vi "GUI_HTT_MultiCamDriveExperiment2.vi"() -> ()   [LabVIEW 2020]
uses:
  Shared/GUI_Template/GUI_master/tcp_new_data_event.ctl
  Shared/GUI_Template/GUI_master/tcp new data cluster.ctl
  General GUIs/Device GUIs/GUI_Cameras/Controls/Crosshair type def.ctl
  <userlib>/_OpenG.lib/array/array.llb/Filter 1D Array with Scalar (String)__ogtk.vi
panel:
  out "String 3":string="x1\ny1\nx2\ny2"
  out "String 2":string="x1\ny1\nx2\ny2"
  out "String":string="x1\ny1\nx2\ny2"
  in  "visibility":bool=TRUE
  out "appended array":string[](array[string]) caption="XH"
  out "appended array 6":string[](array[string]) caption="XH"
  out "appended array 4":string[](array[string]) caption="XH"
  in  "UDP error message":string
  out "tcp data event 2":T1
  out "error IO 2":errorcluster
  in  "Color Box":u32(colorbox)
  in  "TargetSize.Y::4":dbl=45.0 caption="y" min=2.0 max=3000.0 format="%#_6f"
  in  "TargetSize.X::4":dbl=47.0 caption="x" min=2.0 max=3000.0 format="%#_6f"
  in  "TargetSize.Y::3":dbl=163.0 caption="y" min=2.0 max=3000.0 format="%#_6f"
  in  "TargetSize.X::3":dbl=152.0 caption="x" min=2.0 max=3000.0 format="%#_6f"
  in  "TargetSize.Y::2":dbl=74.0 caption="y" min=2.0 max=3000.0 format="%#_6f"
  in  "TargetSize.X::2":dbl=75.0 caption="x" min=2.0 max=3000.0 format="%#_6f"
  in  "active cams":string
  out "CCDs":string[](array[string])
  out "Cameras":T2
  in  "Target.Y::4":dbl=45.0 caption="y" min=0.0 max=2000.0 format="%#_6f"
  in  "Target.X::4":dbl=47.0 caption="x" min=0.0 max=2000.0 format="%#_6f"
  in  "Target.Y::3":dbl=163.0 caption="y" min=0.0 max=2000.0 format="%#_6f"
  in  "Target.X::3":dbl=152.0 caption="x" min=0.0 max=2000.0 format="%#_6f"
  in  "Target.Y::2":dbl=74.0 caption="y" min=0.0 max=2000.0 format="%#_6f"
  in  "Target.X::2":dbl=75.0 caption="x" min=0.0 max=2000.0 format="%#_6f"
  out "error out":errorcluster
  in  "triggerdelay::4":dbl=0.001 caption="triggerdelay" min=0.0 max=10000000.0 format="%_4p"
  in  "triggerdelay::3":dbl=0.001 caption="triggerdelay" min=0.0 max=10000000.0 format="%_4p"
  in  "triggerdelay::2":dbl=0.001 caption="triggerdelay" min=0.0 max=1000000.0 format="%_4p"
  in  "centroidy::5":dbl=0.001 caption="centroid y" min=0.0 max=0.0 format="%_4f"
  in  "centroidx::5":dbl=0.001 caption="centroid x" min=0.0 max=0.0 format="%_4f"
  in  "trigger::4":bool caption="Trigger"
  in  "centroidy::4":dbl=0.001 caption="centroid y" min=0.0 max=0.0 format="%_4f"
  in  "centroidx::4":dbl=0.001 caption="centroid x" min=0.0 max=0.0 format="%_4f"
  in  "exposure::4":dbl=0.001 caption="exposure" min=0.0001 max=100000.0 format="%_4p"
  out "image::4":T3(plugin-control) caption="HTT-MagCam-02"
  in  "GUIdevice 4":string="HTT-C14_3_topjet"
  in  "trigger::3":bool caption="Trigger"
  in  "centroidy::3":dbl=0.001 caption="centroid y" min=0.0 max=0.0 format="%_4f"
  in  "centroidx::3":dbl=0.001 caption="centroid x" min=0.0 max=0.0 format="%_4f"
  in  "exposure::3":dbl=0.001 caption="exposure" min=1.0 max=10000000.0 format="%_4p"
  out "image::3":T3(plugin-control) caption="HTT-MagCam-03"
  in  "GUIdevice 3":string="HTT-C26_1_ppoint2"
  in  "trigger::2":bool caption="Trigger"
  in  "centroidy::2":dbl=0.001 caption="centroid y" min=0.0 max=0.0 format="%_4f"
  in  "centroidx::2":dbl=0.001 caption="centroid x" min=0.0 max=0.0 format="%_4f"
  in  "exposure::2":dbl=0.001 caption="exposure" min=0.0001 max=1.0 format="%_4p"
  out "image::2":T3(plugin-control) caption="HTT-MagCam-04"
  in  "GUIdevice 2":string="HTT-C14_2_if"
  out "tcp data event":T1
  in  "Refresh Button":bool caption="Update Crosshairs"
  in  "Select device":string(combo)="FrogHPD"
  in  "stop":bool
  in  "GUIdevice 1":string="HPD_CCD"
  # "XHair location"
  # "XHair location"
  # "XHair size"
  # "XHair size"
  # "XHair location"
  # "XHair size"
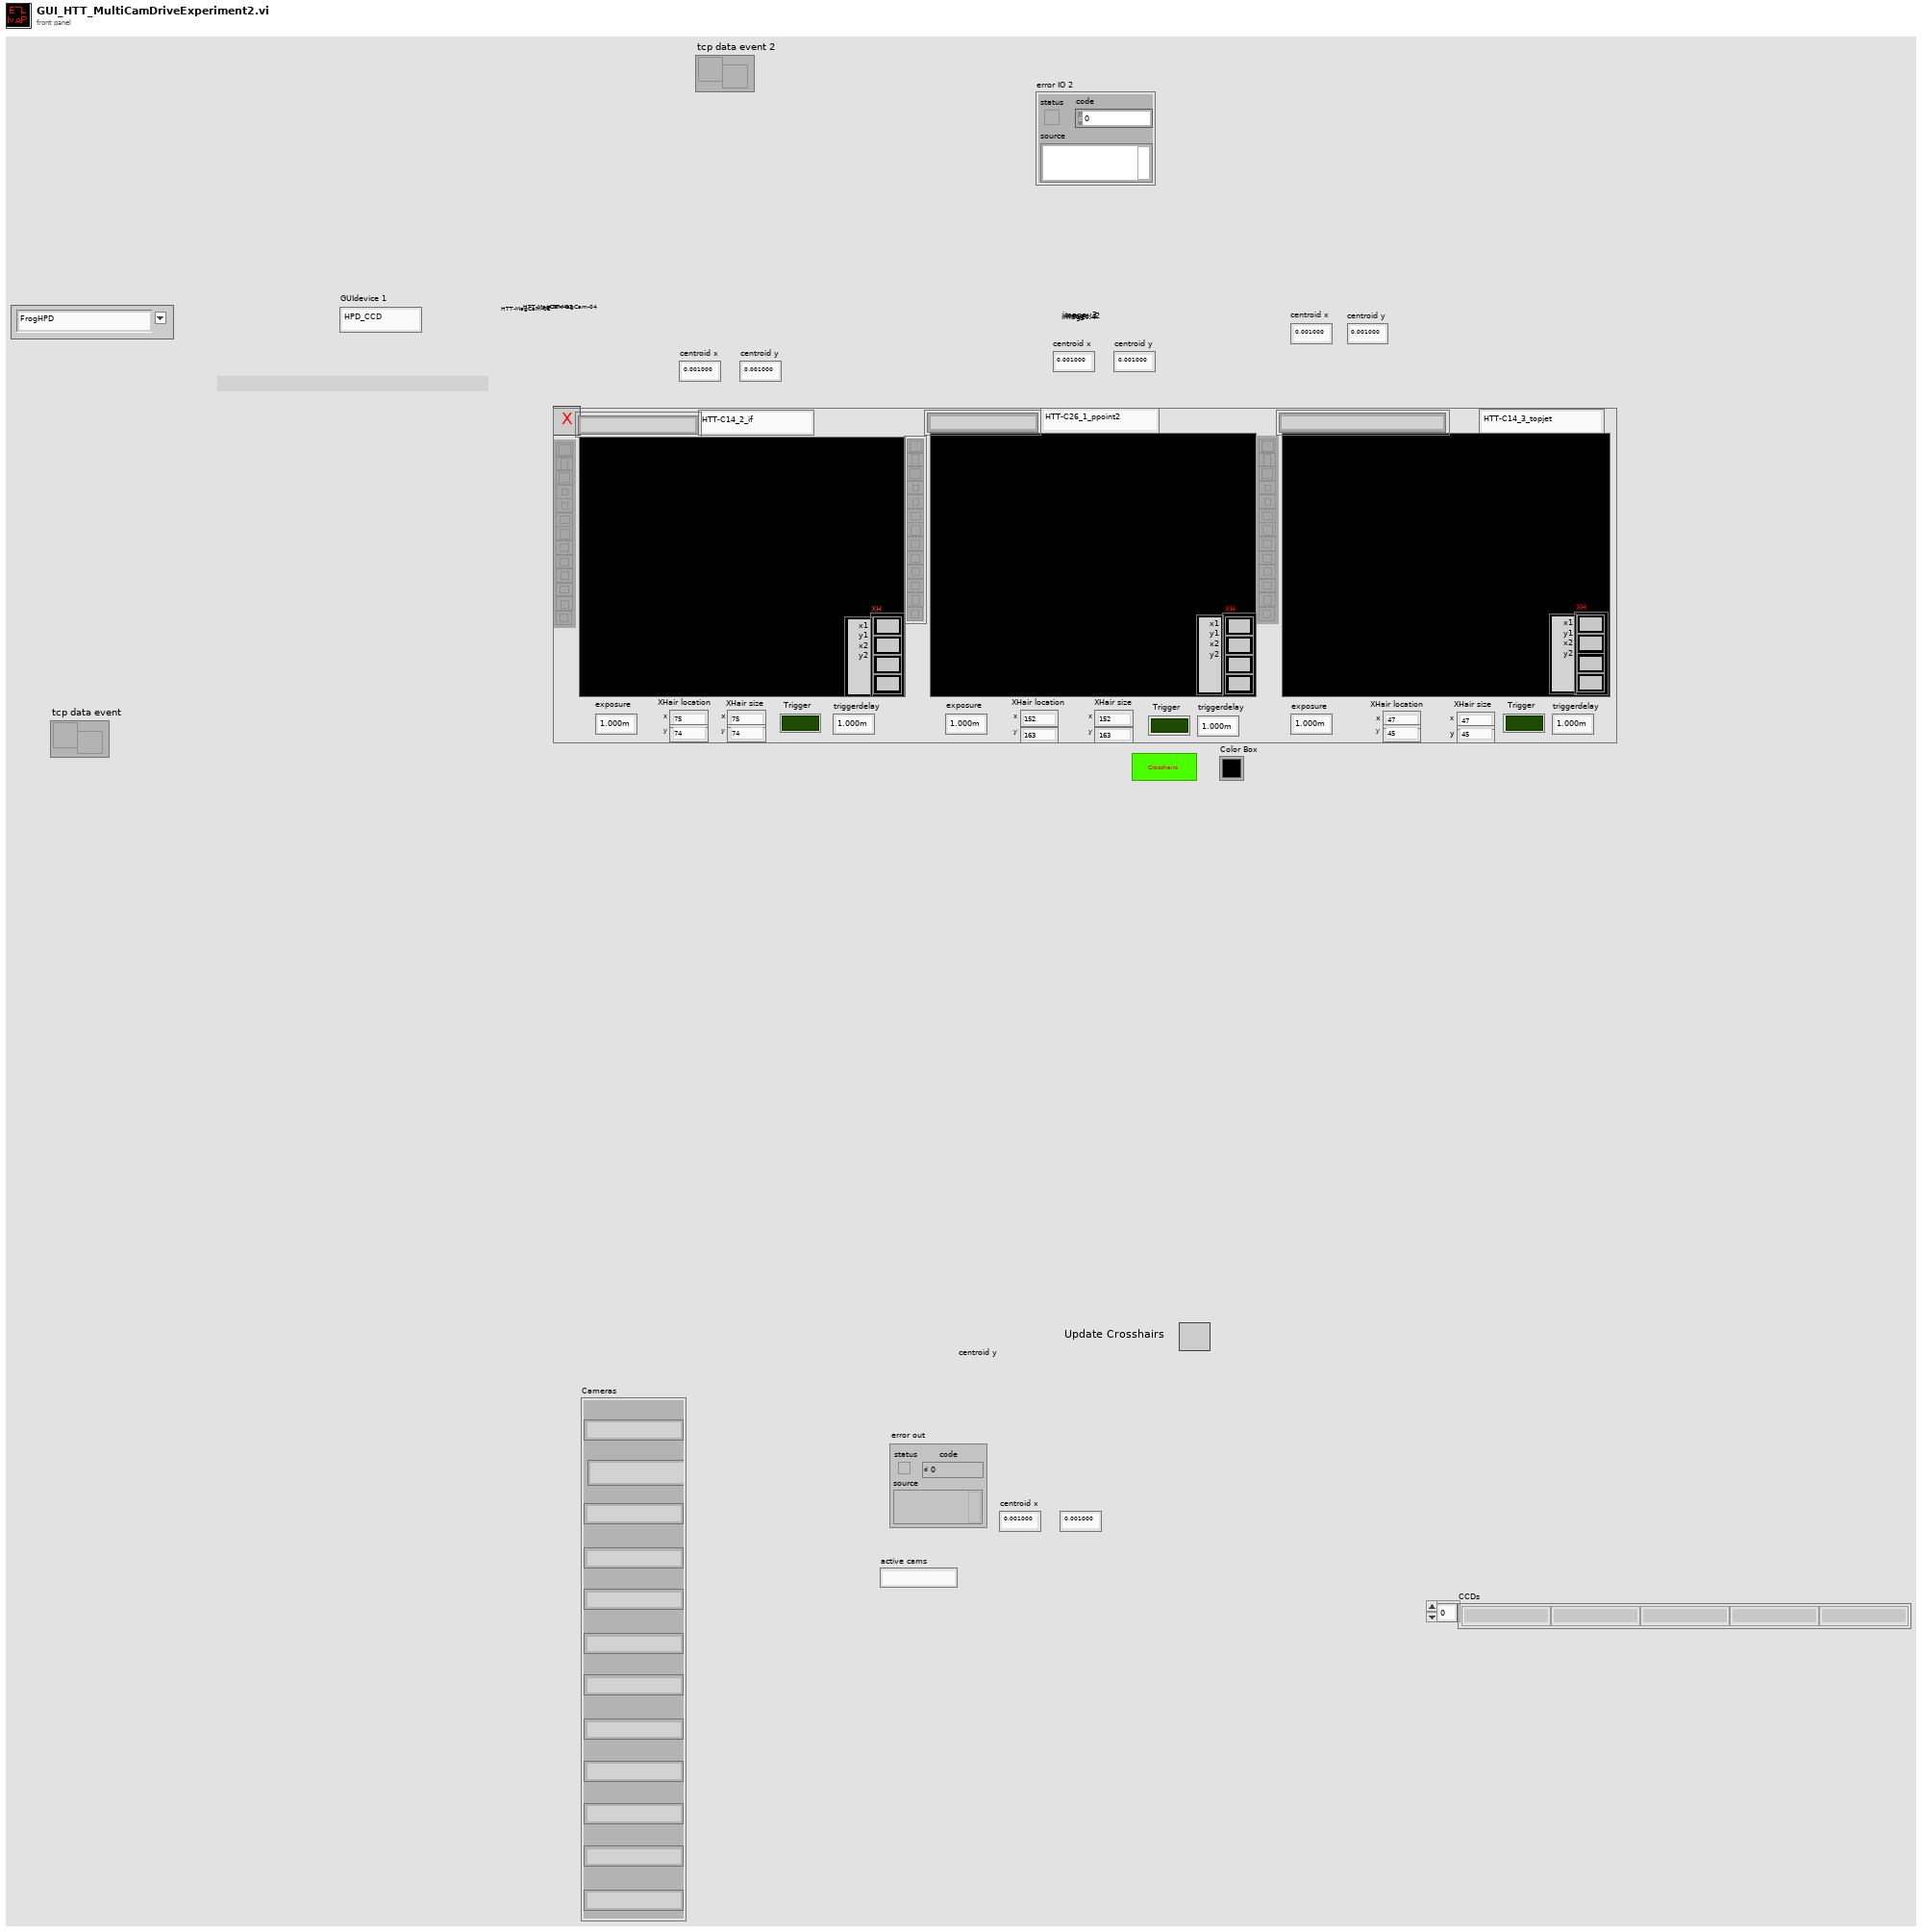
[diagram p1: front panel]
types:
  T1 = typedef "tcp_new_data_event.ctl" = refnum<user-event>
  T2 = cluster{"[0]":string, "[1]":string, "[2]":string, "[3]":string, "[4]":string, "[5]":string, "[6]":string, "[7]":string, "[8]":string, "[8] 2":string, "[8] 3":string, "[8] 4":string}
  T3 = typedef "IMAQ Image.ctl" = refnum<image>
  T4 = typedef "Image Type" = u32
  T5 = cluster{"Target.X::2":refnum<vi>, "Target.Y::2":refnum<vi>}
  T6 = cluster{"Target.X::3":refnum<vi>, "Target.Y::3":refnum<vi>}
  T7 = cluster{"Target.X::4":refnum<vi>, "Target.Y::4":refnum<vi>}
  T8 = cluster{"TargetSize.X::2":refnum<vi>, "TargetSize.Y::2":refnum<vi>}
  T9 = cluster{"TargetSize.X::3":refnum<vi>, "TargetSize.Y::3":refnum<vi>}
  T10 = cluster{"TargetSize.X::4":refnum<vi>, "TargetSize.Y::4":refnum<vi>}
  T11 = cluster{"Target.X::4":refnum<vi>, "Target.Y::4":refnum<vi>}[]
  T12 = cluster{"TargetSize.X::4":refnum<vi>, "TargetSize.Y::4":refnum<vi>}[]
  T13 = cluster{"[0]":string, "[1]":string, "[2]":string, "[3]":string, "[4]":string, "[5]":string, "[6]":string, "[7]":string, "[8]":string, "[9]":string, "[10]":string, "[11]":string}
  T14 = typedef "Crosshair type def.ctl" = cluster{"Draw":bool, "Target":cluster{"x":dbl, "y":dbl}, "Size":cluster{"x":dbl, "y":dbl}, "Angle":dbl, "Color":u32, "Thickness":u8, "CrosshairLabel":string}
  T15 = cluster{"Left":i32, "Top":i32, "Right":i32, "Bottom":i32}
  T16 = enum32{"invalid app kind", "Development System", "Run Time System", "Student Edition", "Embedded LabVIEW", "Evaluation", "Custom"}
  T17 = typedef "tcp new data cluster.ctl" = cluster{"EventEnum":enum16{"new data", "connection status update"}, "Device name":string}
  T18 = enum32{"Invalid", "Standard", "Closed", "Hidden", "Minimized", "Maximized"}
  T19 = cluster{"Core":cluster{"Current VI Reference":refnum<vi>, "Close Panel on Exit?":bool}, "Your Boolean data":bool, "active cams":string, "SuperGUI":cluster{"STOP queue":refnum<queue>, "SuperGUI ref":refnum<vi>}}
  T20 = cluster{"STOP queue":refnum<queue>, "SuperGUI ref":refnum<vi>}
  T21 = cluster{"Current VI Reference":refnum<vi>, "Close Panel on Exit?":bool}
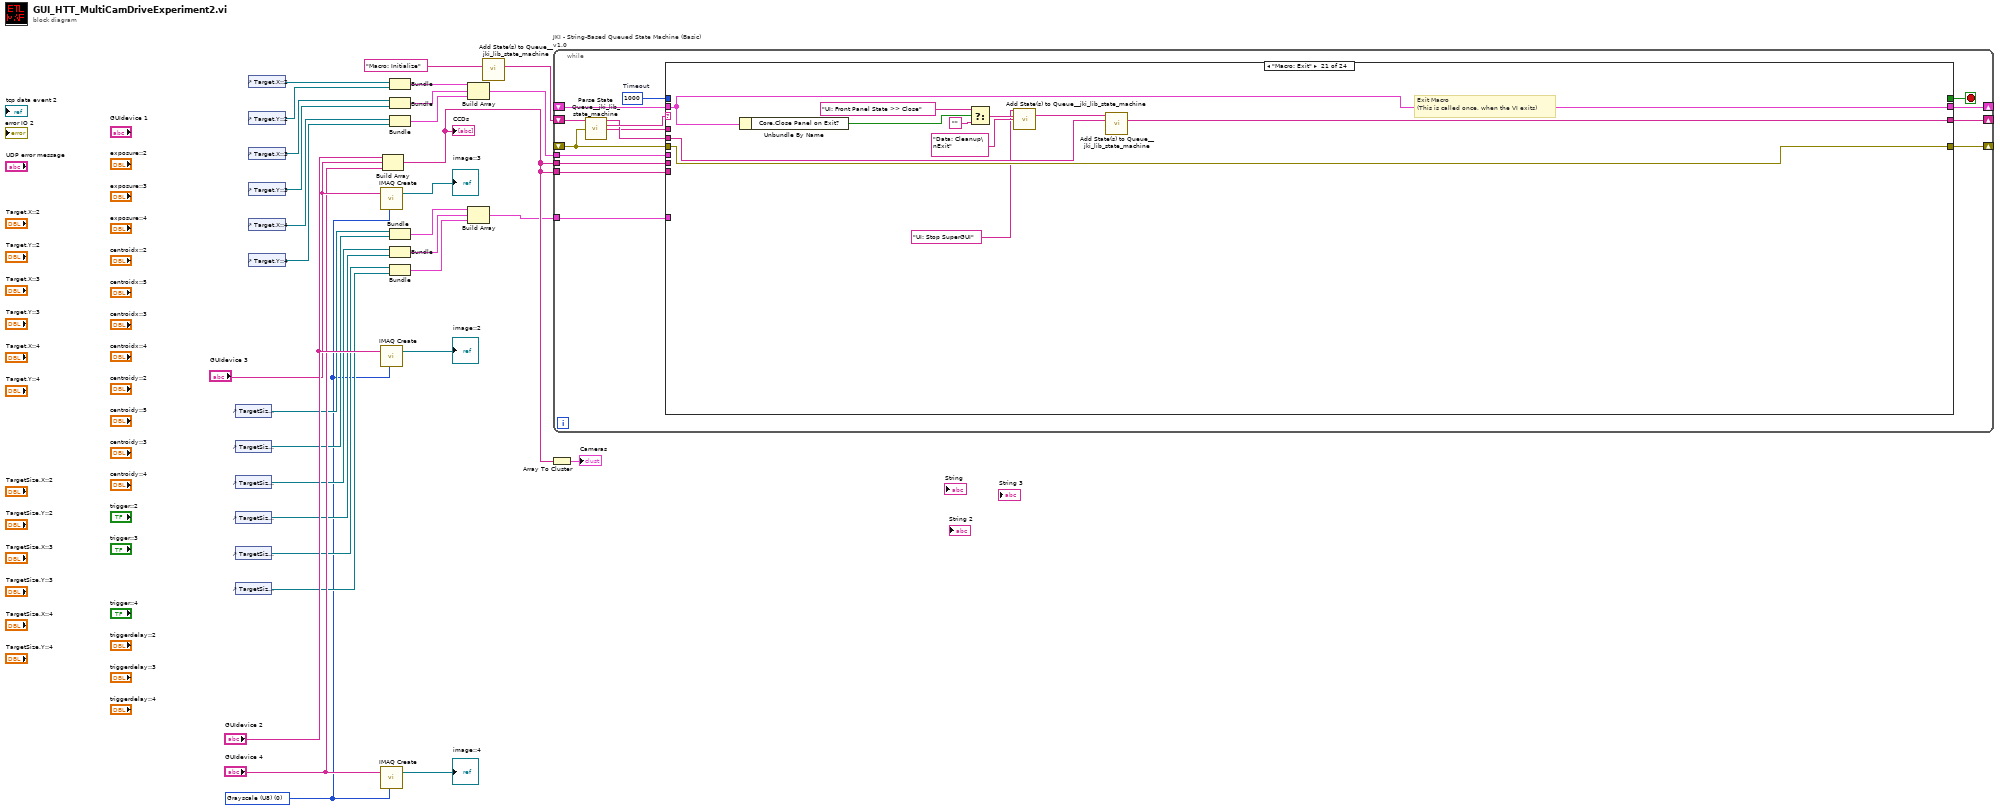
[diagram p0: block diagram]
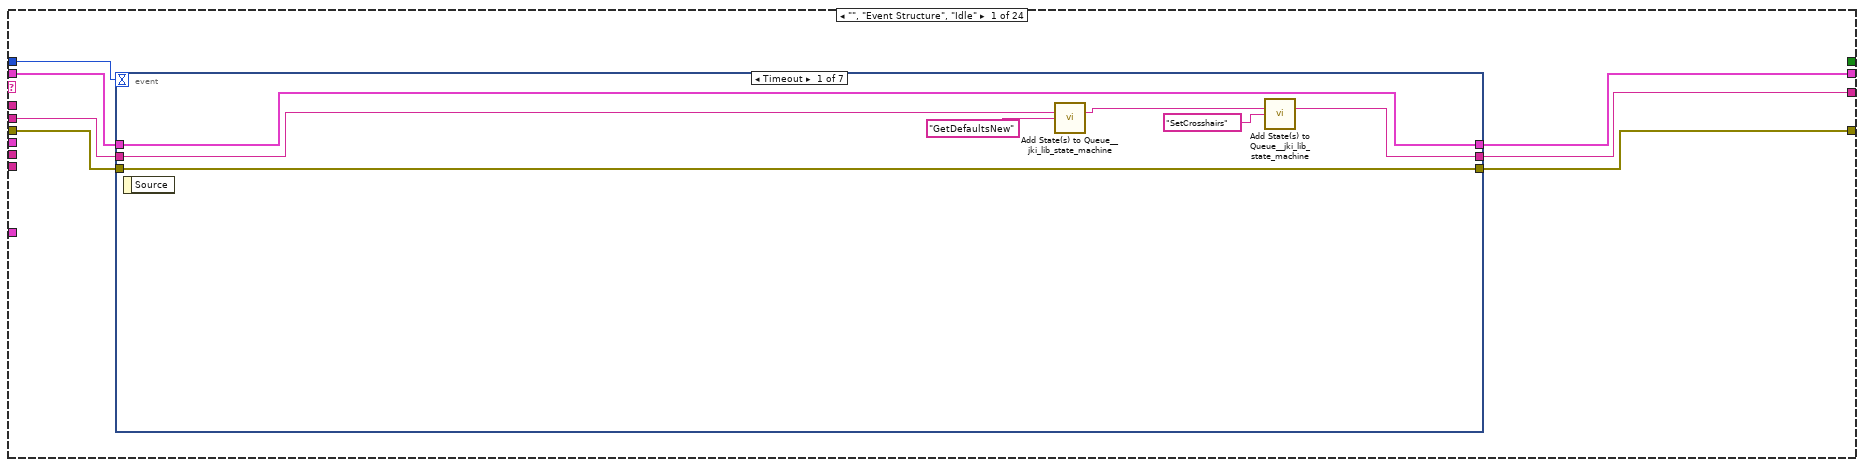
[diagram p2: hidden frame]
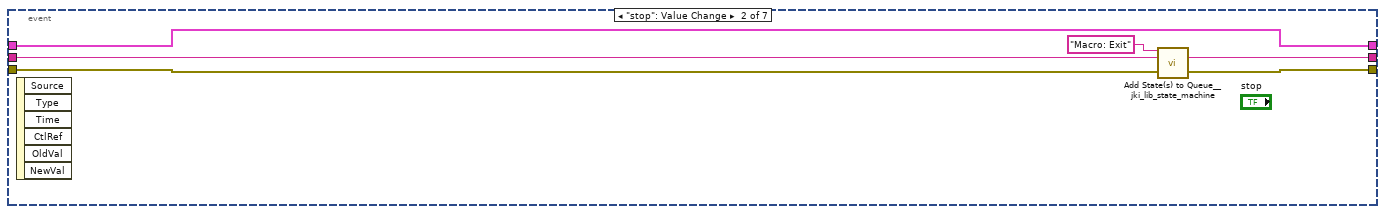
[diagram p3: hidden frame]
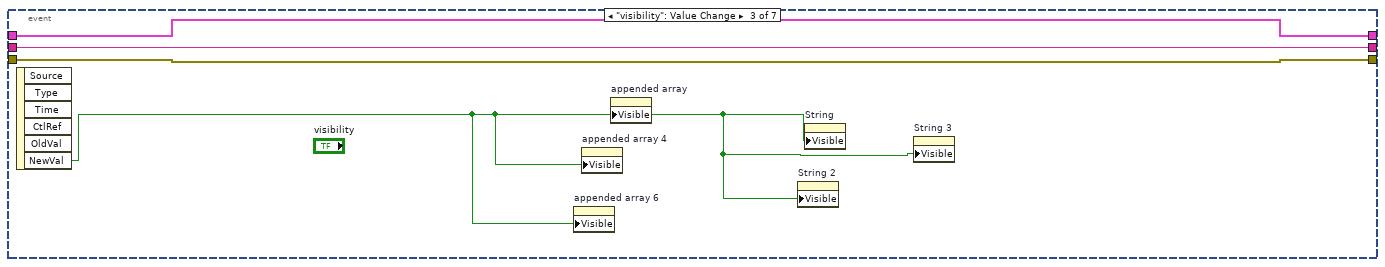
[diagram p4: hidden frame]
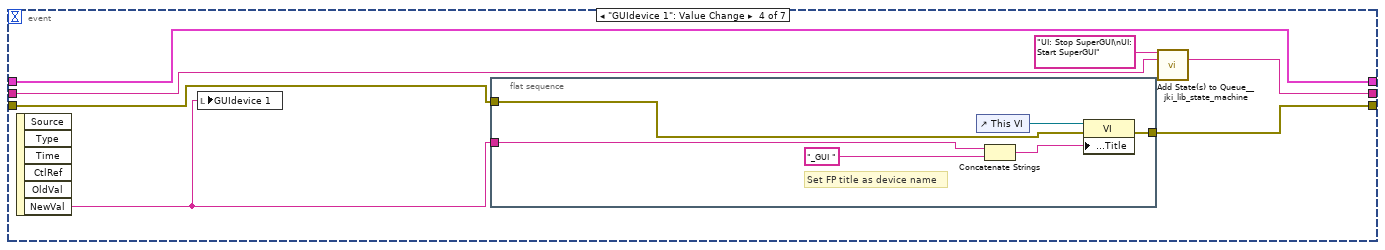
[diagram p5: hidden frame]
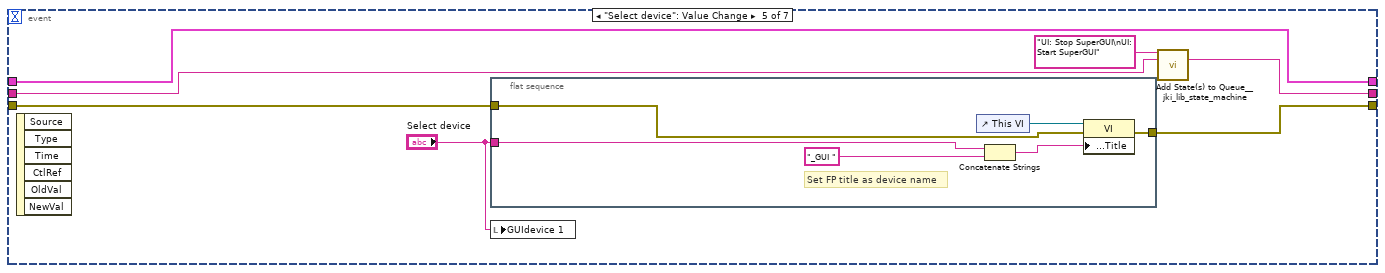
[diagram p6: hidden frame]
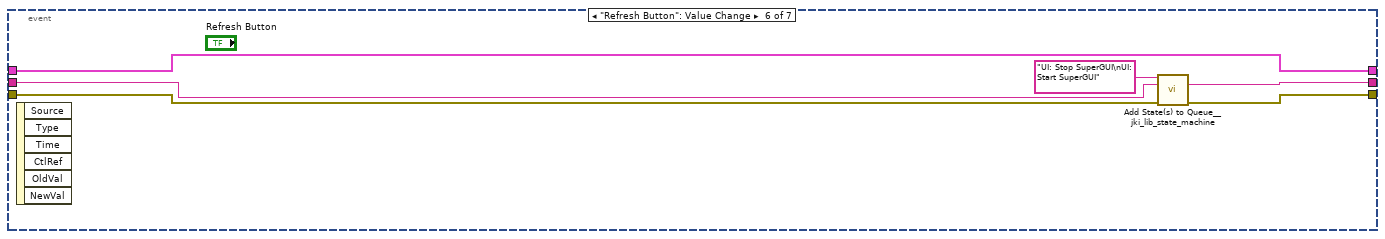
[diagram p7: hidden frame]
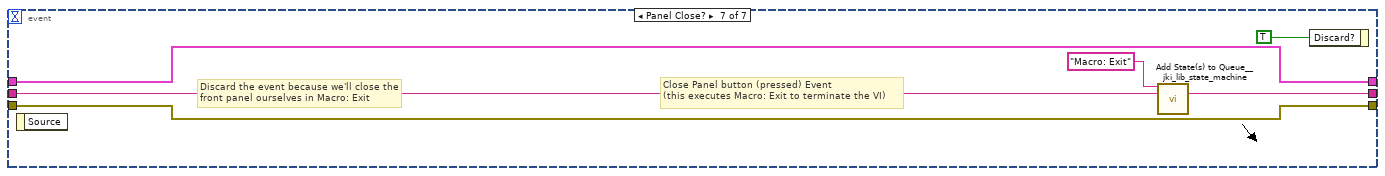
[diagram p8: hidden frame]
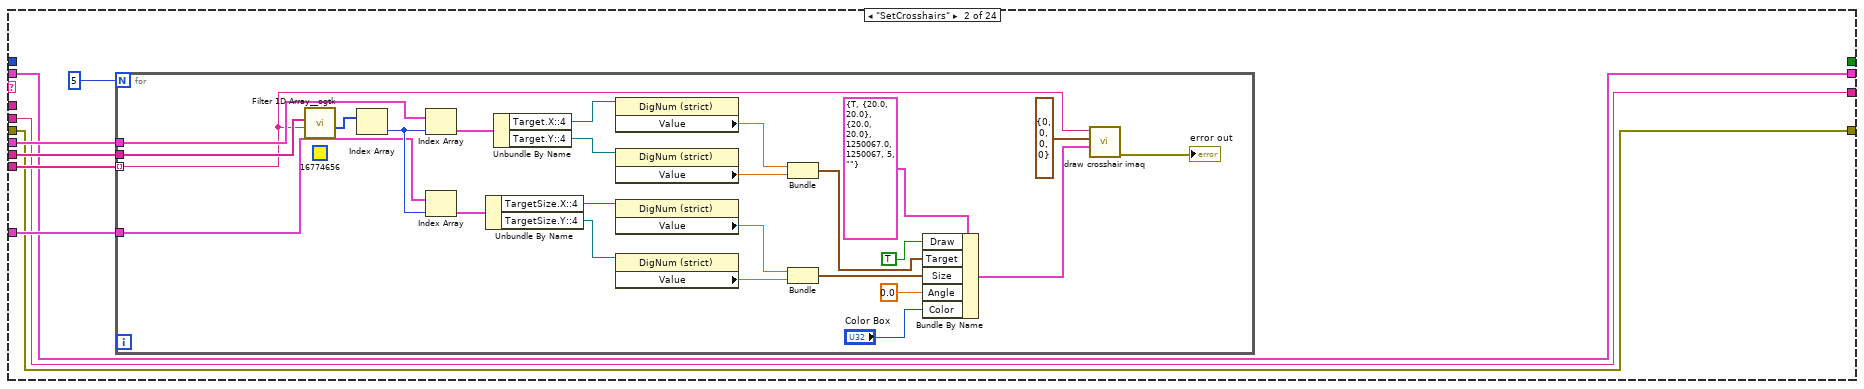
[diagram p9: hidden frame]
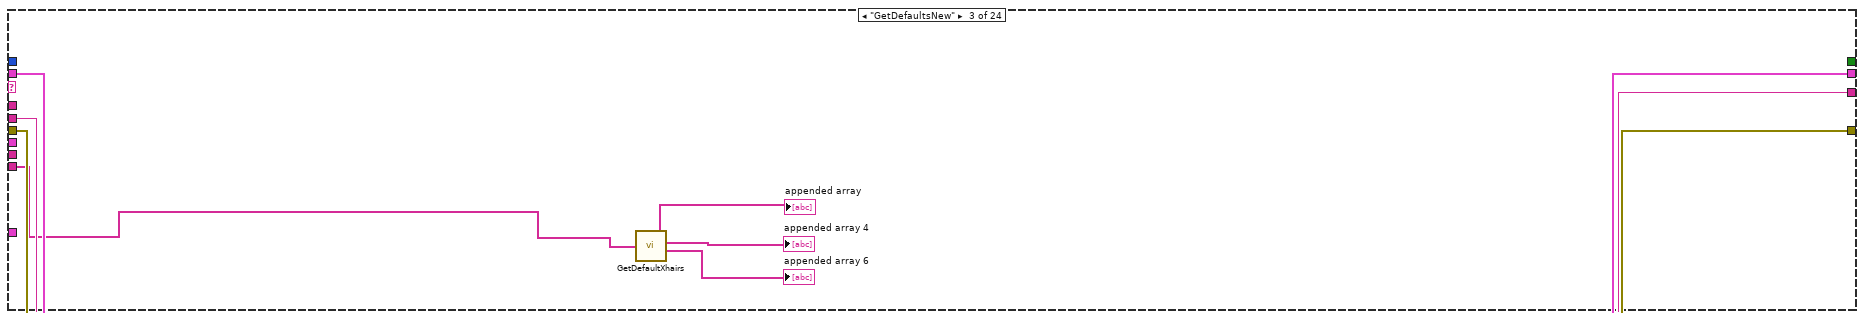
[diagram p10: hidden frame]
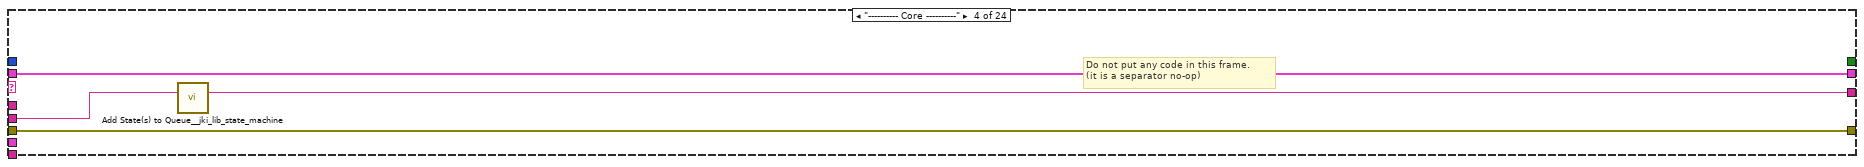
[diagram p11: hidden frame]
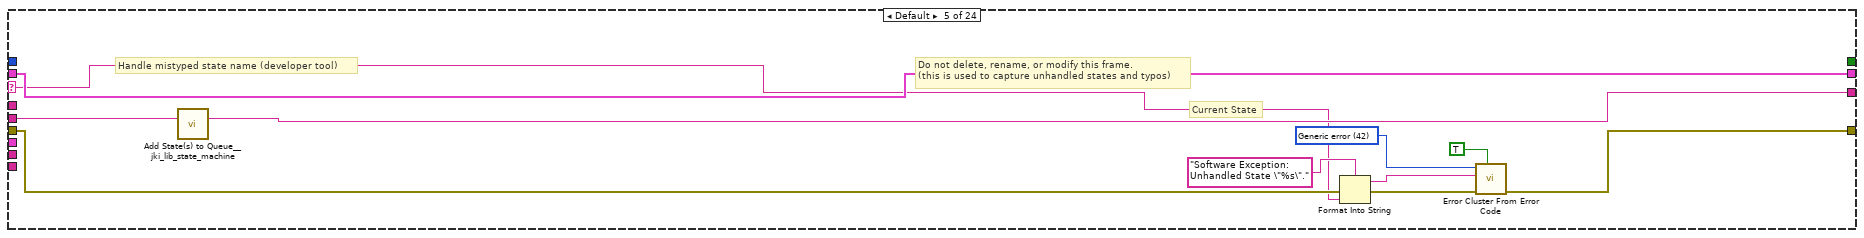
[diagram p12: hidden frame]
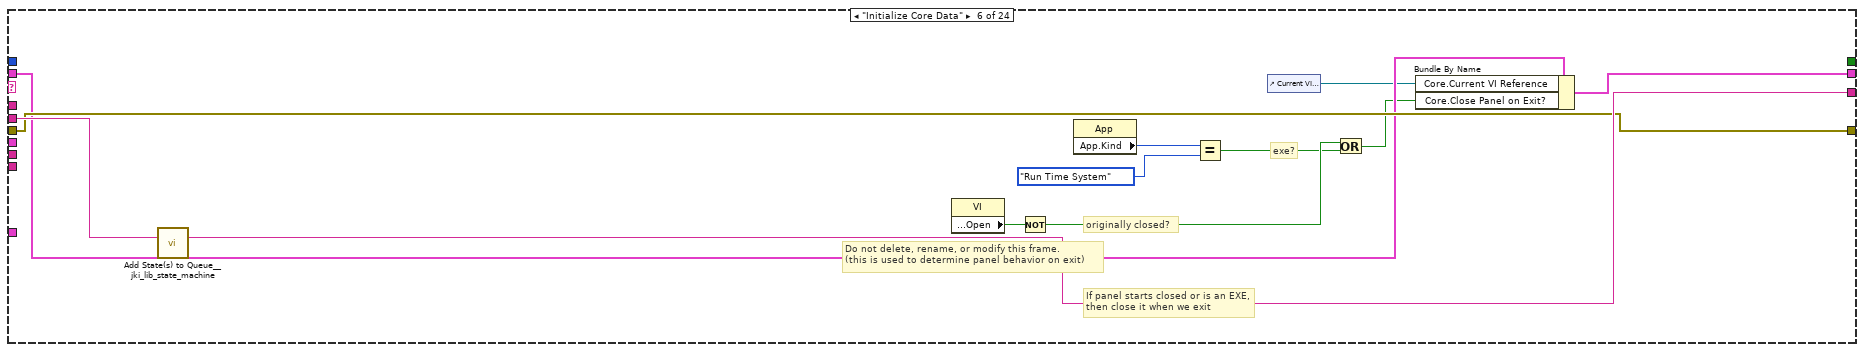
[diagram p13: hidden frame]
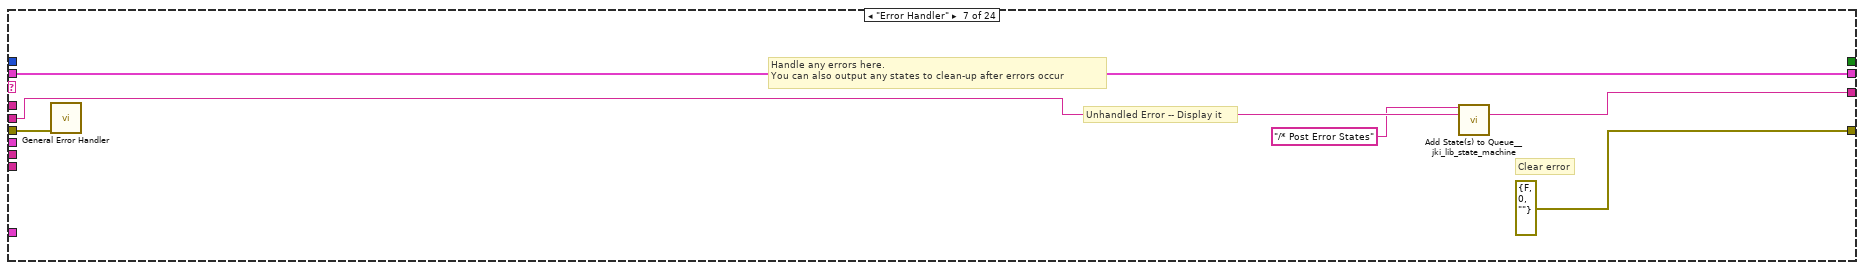
[diagram p14: hidden frame]
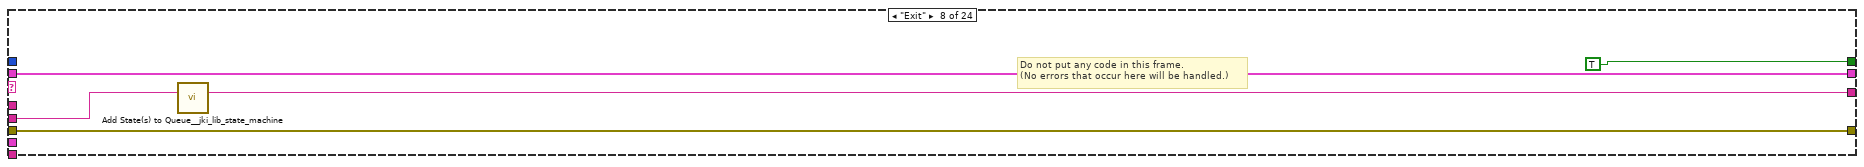
[diagram p15: hidden frame]
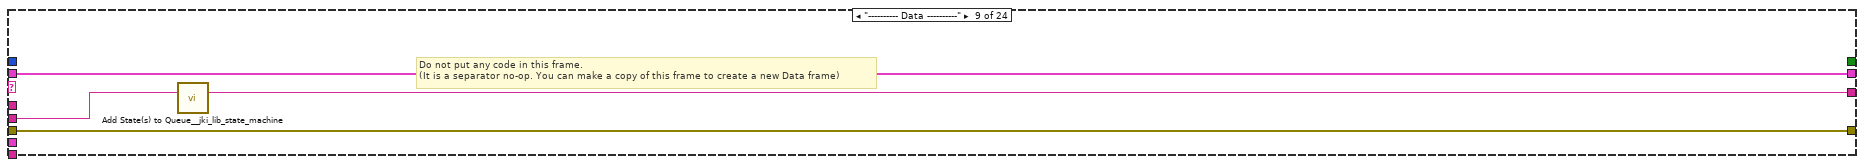
[diagram p16: hidden frame]
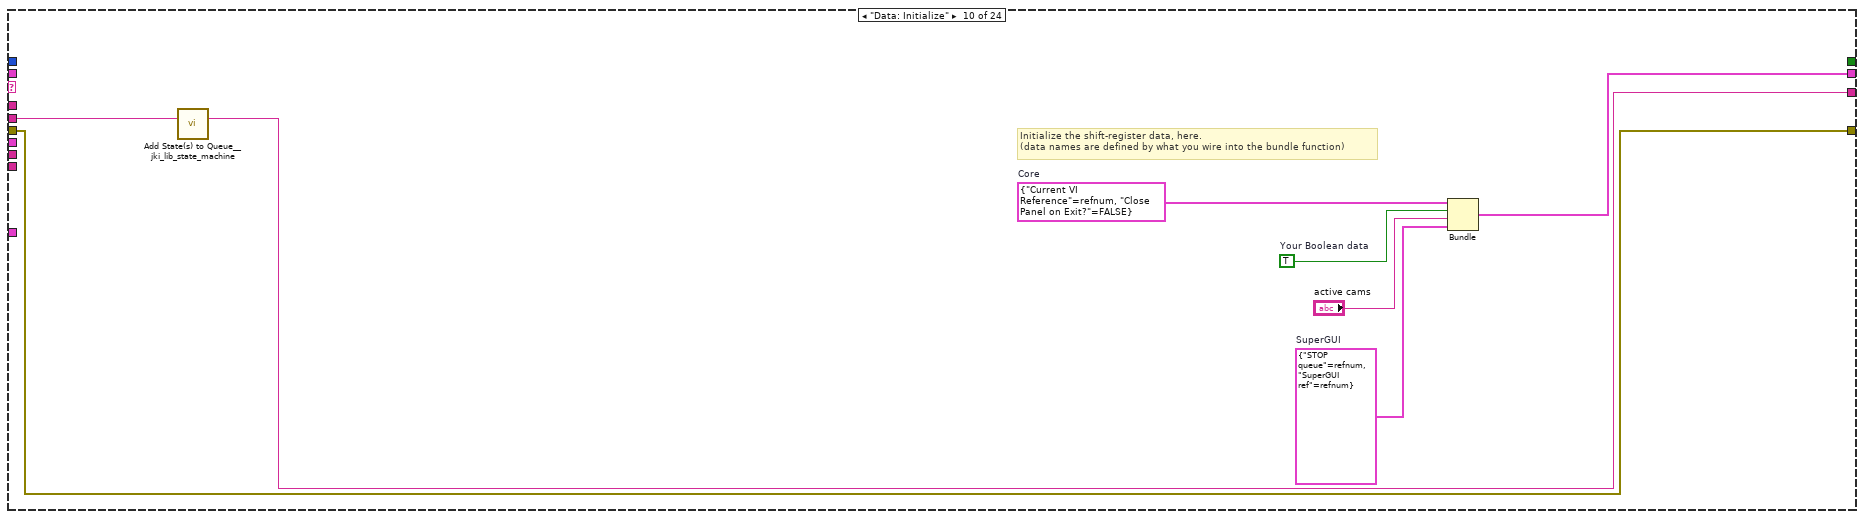
[diagram p17: hidden frame]
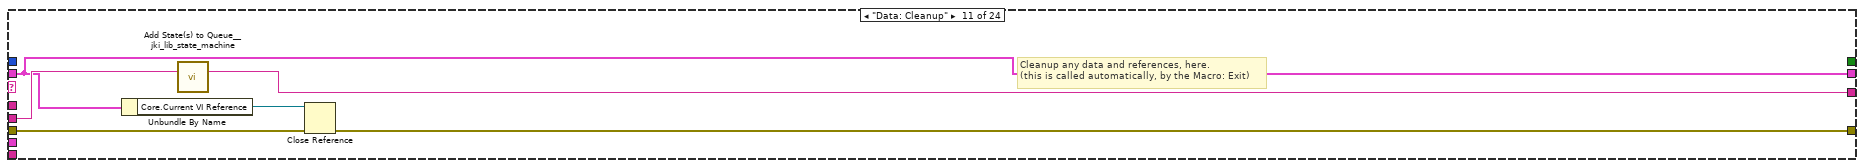
[diagram p18: hidden frame]
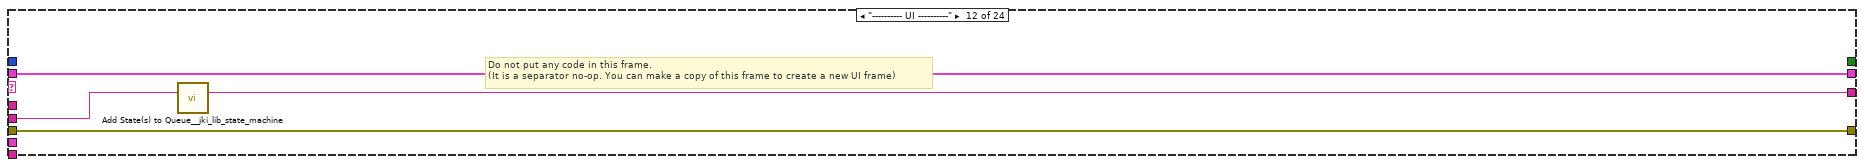
[diagram p19: hidden frame]
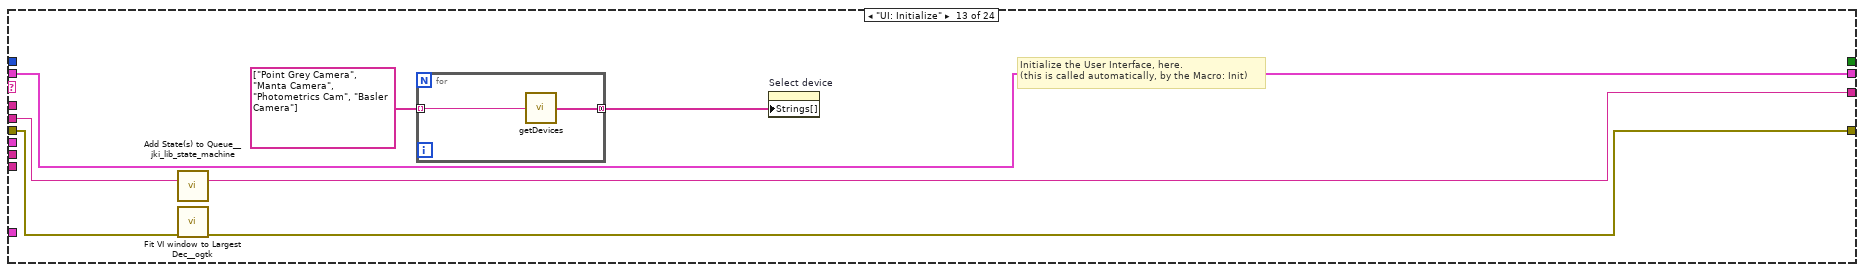
[diagram p20: hidden frame]
diagram:
  w1 = T4 0 items=["Grayscale (U8)", "Grayscale (I16)", "Grayscale (SGL)", "Complex (CSG)", "RGB (U32)", "HSL (U32)", "RGB (U64)", "Grayscale (U16)"] ("Image Type")
  n1 = control-ref of="TargetSize.X::2"() -> (w11:refnum<vi>)
  n2 = control-ref of="TargetSize.Y::2"() -> (w10:refnum<vi>)
  n3 = control-ref of="TargetSize.X::3"() -> (w9:refnum<vi>)
  n4 = control-ref of="TargetSize.Y::3"() -> (w8:refnum<vi>)
  n5 = control-ref of="TargetSize.X::4"() -> (w7:refnum<vi>)
  n6 = control-ref of="TargetSize.Y::4"() -> (w6:refnum<vi>)
  n7 = control-ref of="Target.X::2"() -> (w26:refnum<vi>)
  n8 = control-ref of="Target.Y::2"() -> (w25:refnum<vi>)
  n9 = control-ref of="Target.X::3"() -> (w24:refnum<vi>)
  n10 = control-ref of="Target.Y::3"() -> (w23:refnum<vi>)
  n11 = control-ref of="Target.X::4"() -> (w22:refnum<vi>)
  n12 = control-ref of="Target.Y::4"() -> (w21:refnum<vi>)
  n13 = call "IMAQ Create"("Image Name"="GUIdevice 3", "Image Type"=w1) -> ("New Image"=→"image::3":T3)  [unwired: 3 in, 1 out]
  n14 = call "IMAQ Create"("Image Name"="GUIdevice 2", "Image Type"=w1) -> ("New Image"=→"image::2":T3)  [unwired: 3 in, 1 out]
  n15 = call "IMAQ Create"("Image Name"="GUIdevice 4", "Image Type"=w1) -> ("New Image"=→"image::4":T3)  [unwired: 3 in, 1 out]
  n16 = Build Array("GUIdevice 2", "GUIdevice 3", "GUIdevice 4") -> (w12:string[])
  "CCDs" <- w12
  n17 = Bundle("Target.X::2"=w26, "Target.Y::2"=w25) -> (w20:T5)  [unwired: 1 in]
  n18 = Bundle("Target.X::3"=w24, "Target.Y::3"=w23) -> (w19:T6)  [unwired: 1 in]
  n19 = Bundle("Target.X::4"=w22, "Target.Y::4"=w21) -> (w18:T7)  [unwired: 1 in]
  n20 = Bundle("TargetSize.X::2"=w11, "TargetSize.Y::2"=w10) -> (w5:T8)  [unwired: 1 in]
  n21 = Bundle("TargetSize.X::3"=w9, "TargetSize.Y::3"=w8) -> (w4:T9)  [unwired: 1 in]
  n22 = Bundle("TargetSize.X::4"=w7, "TargetSize.Y::4"=w6) -> (w3:T10)  [unwired: 1 in]
  n23 = Build Array(w20, w19, w18) -> (w17:T11)
  n24 = Build Array(w5, w4, w3) -> (w2:T12)
  n25 = call <vilib>:"Add State(s) to Queue__jki_lib_state_machine.vi"("State(s) in (\"\")"="Macro: Initialize") -> ("States Out"=w31:string)  [unwired: 14 in]
  n26 = Array To Cluster(array=w12) -> (cluster=→"Cameras":T13)
  n27 = while "JKI - String-Based Queued State Machine (Basic) v1.0" {
    shift-right: [w39] -> _
    shift-left: _ -> [w36]
    shift-right: [w42] -> _
    shift-left: _ -> [w37]
    shift-right: [w41] -> _
    shift-left: w31 -> [w43]
    tunnel: w17 -> [w33]
    tunnel: w12 -> [w34]
    tunnel: w12 -> [w35]
    tunnel: w2 -> [w32]
    stop <- w40 stop-if-true
    w38 = 1000  # Timeout
    n28 = call <vilib>:"Parse State Queue__jki_lib_state_machine.vi"("State Queue"=w43, "Error In (no error)"=w37) -> ("Remaining States"=w45:string, "Current State"=w46:string, "Arguments"=w44:string)  [unwired: 11 in]
    n29 = case shown="\"Macro: Exit\"" w46 {
      selector: w46 -> [_ _ _ _ w151 _ _ _ _ _ _ _ _ _ _ _ _ _ _ _ _ _ _ _]
      tunnel: w45 -> [w53 w109 w145 w150 w155 w173 w179 w184 w188 w196 w202 w206 w213 w221 w256 w264 w270 w281 w307 w312 w323 w327 w331 w335]
      tunnel: w44 -> [_ _ _ _ _ _ _ _ _ _ _ _ _ _ _ _ w265 w275 _ _ _ _ _ _]
      tunnel: w36 -> [w51 w110 w146 w147 w153 w164 w176 w182 w185 _ w197 w203 w211 w219 w247 w259 w268 w277 w304 w309 w320 w324 w328 w332]
      tunnel: [w50 w108 w144 w148 w157 w170 errorcluster {"status"=FALSE, "code"=0, "source"=""} ("error out") w181 w186 w193 w198 w204 w209 w216 w240 w257 w266 w278 w305 w310 w321 w325 w329 w333] -> w42
      tunnel: w37 -> [w49 w108 w144 w148 w156 w170 w175 w181 w186 w193 w199 w204 w210 w217 w241 w258 w267 w279 w305 w310 w321 w325 w329 w333]
      tunnel: [w52 w109 w145 w149 w154 w172 w178 w183 w187 w195 w201 w205 w212 w220 w255 w263 w269 w280 w306 w311 w322 w326 w330 w334] -> w41
      tunnel: [_ _ _ _ _ _ _ TRUE _ _ _ _ _ _ _ _ _ _ _ _ _ _ _ _] -> w40
      tunnel: [w48 w110 w146 w147 w153 w171 w176 w182 w185 w194 w197 w203 w211 w219 w246 w259 w268 w277 w304 w309 w320 w324 w328 w332] -> w39
      tunnel: w38 -> [w47 _ _ _ _ _ _ _ _ _ _ _ _ _ _ _ _ _ _ _ _ _ _ _]
      tunnel: w35 -> [_ w112 w143 _ _ _ _ _ _ _ _ _ _ _ _ _ _ _ _ _ _ _ _ _]
      tunnel: w34 -> [_ w113 _ _ _ _ _ _ _ _ _ _ _ _ _ _ _ _ _ _ _ _ _ _]
      tunnel: w33 -> [_ w114 _ _ _ _ _ _ _ _ _ _ _ _ _ _ _ _ _ _ _ _ _ _]
      tunnel: w32 -> [_ w111 _ _ _ _ _ _ _ _ _ _ _ _ _ _ _ _ _ _ _ _ _ _]
      frame "", "Event Structure", "Idle" {
        n30 = event shown="[0] Timeout" {
          selector: _ -> [_ _ _ _ _ _ _]
          dyn-events: _ -> [_ _ _ _ _ _ _]
          timeout: w47 -> [_ _ _ _ _ _ _]
          tunnel: w53 -> [w56 w63 w67 w73 w85 w98 w106]
          tunnel: [w60 w62 w67 w72 w84 w97 w105] -> w52
          tunnel: w51 -> [w58 w65 w69 w76 w89 w100 w103]
          tunnel: [w59 w64 w68 w74 w87 w99 w104] -> w50
          tunnel: w49 -> [w59 w64 w68 w75 w88 w99 w104]
          tunnel: [w58 w65 w69 w76 w89 w100 w103] -> w48
          event Timeout {
            n31 = event-data() -> ()  [unwired: 1 in, 1 out]
            n32 = call <vilib>:"Add State(s) to Queue__jki_lib_state_machine.vi"("State(s) in (\"\")"=w56, "State(s) at Back (\"\")"="GetDefaultsNew") -> ("States Out"=w54:string)  [unwired: 13 in]
            n33 = call <vilib>:"Add State(s) to Queue__jki_lib_state_machine.vi"("State(s) in (\"\")"=w54, "State(s) at Back (\"\")"="SetCrosshairs") -> ("States Out"=w60:string)  [unwired: 13 in]
          }
          event "stop": Value Change {
            n34 = event-data() -> ()  [unwired: 1 in, 6 out]
            n35 = call <vilib>:"Add State(s) to Queue__jki_lib_state_machine.vi"("State(s) in Front (\"\")"="Macro: Exit", "State(s) in (\"\")"=w63) -> ("States Out"=w62:string)  [unwired: 13 in]
          }
          event "visibility": Value Change {
            n36 = event-data() -> ("NewVal"=w66:bool)  [unwired: 1 in, 5 out]
            n37 = property on="appended array 6" class="Arr (strict)"("Visible"=w66) -> ()  [unwired: 2 in, 2 out]
            n38 = property on="appended array 4" class="Arr (strict)"("Visible"=w66) -> ()  [unwired: 2 in, 2 out]
            n39 = property on="appended array" class="Arr (strict)"("Visible"=w66) -> ()  [unwired: 2 in, 2 out]
            n40 = property on="String 2" class="Str"("Visible"=w66) -> ()  [unwired: 2 in, 2 out]
            n41 = property on="String" class="Str"("Visible"=w66) -> ()  [unwired: 2 in, 2 out]
            n42 = property on="String 3" class="Str"("Visible"=w66) -> ()  [unwired: 2 in, 2 out]
          }
          event "GUIdevice 1": Value Change {
            n43 = event-data() -> ("NewVal"=w70:string)  [unwired: 1 in, 5 out]
            n44 = local write "GUIdevice 1"(w70) -> ()
            n45 = flat-sequence {
              tunnel: [w79] -> w74
              tunnel: w75 -> [w78]
              tunnel: w70 -> [w77]
              frame #0 {
                # "Set FP title as device name"
                n46 = control-ref of="This VI"() -> (w82:refnum<vi>)
                n47 = Concatenate Strings(w77, "_GUI ") -> (w81:string)
                n48 = property class="VI"(reference=w82, error in=w78, "Front Panel.Title"=w81) -> (error out=w79:errorcluster)  [unwired: 1 out]
              }
            }
            n49 = call <vilib>:"Add State(s) to Queue__jki_lib_state_machine.vi"("State(s) in Front (\"\")"="UI: Stop SuperGUI\nUI: Start SuperGUI", "State(s) in (\"\")"=w73) -> ("States Out"=w72:string)  [unwired: 13 in]
          }
          event "Select device": Value Change {
            n50 = event-data() -> ()  [unwired: 1 in, 6 out]
            n51 = flat-sequence {
              tunnel: [w92] -> w87
              tunnel: w88 -> [w91]
              tunnel: "Select device" -> [w90]
              frame #0 {
                # "Set FP title as device name"
                n52 = control-ref of="This VI"() -> (w95:refnum<vi>)
                n53 = Concatenate Strings(w90, "_GUI ") -> (w94:string)
                n54 = property class="VI"(reference=w95, error in=w91, "Front Panel.Title"=w94) -> (error out=w92:errorcluster)  [unwired: 1 out]
              }
            }
            n55 = local write "GUIdevice 1"("Select device") -> ()
            n56 = call <vilib>:"Add State(s) to Queue__jki_lib_state_machine.vi"("State(s) in Front (\"\")"="UI: Stop SuperGUI\nUI: Start SuperGUI", "State(s) in (\"\")"=w85) -> ("States Out"=w84:string)  [unwired: 13 in]
          }
          event "Refresh Button": Value Change {
            n57 = event-data() -> ()  [unwired: 1 in, 6 out]
            n58 = call <vilib>:"Add State(s) to Queue__jki_lib_state_machine.vi"("State(s) in Front (\"\")"="UI: Stop SuperGUI\nUI: Start SuperGUI", "State(s) in (\"\")"=w98) -> ("States Out"=w97:string)  [unwired: 13 in]
          }
          event Panel Close? {
            # "Discard the event because we'll close the front panel ourselves in Macro: Exit"
            # "Close Panel button (pressed) Event\n(this executes Macro: Exit to terminate the VI)"
            n59 = event-data() -> ()  [unwired: 1 in, 1 out]
            n60 = call <vilib>:"Add State(s) to Queue__jki_lib_state_machine.vi"("State(s) in Front (\"\")"="Macro: Exit", "State(s) in (\"\")"=w106) -> ("States Out"=w105:string)  [unwired: 13 in]
            n61 = event-data("Discard?"=TRUE) -> ()  [unwired: 1 in, 1 out]
          }
        }
      }
      frame "SetCrosshairs" {
        n62 = for {
          N: 5 -> [_]
          tunnel: w113 -> [w118]
          tunnel: w114 -> [w117]
          tunnel: w111 -> [w116]
          tunnel: w112 -> [w115] mode=indexing
          (unwired) u32 16774656 ("Color")
          n63 = call-poly <userlib>:"Filter 1D Array__ogtk.vi"("items to filter"=w115, "array"=w118) -> ("filtered item indices"=w122:i32[])  [unwired: 4 in, 1 out]
          n64 = Index Array(array=w122) -> (element=w125:i32)  [unwired: 1 in]
          n65 = Index Array(array=w117, index=w125) -> (element=w123:T7)
          n66 = Index Array(array=w116, index=w125) -> (element=w126:T10)
          n67 = Unbundle By Name(w126) -> ("TargetSize.X::4"=w127:refnum<vi>, "TargetSize.Y::4"=w128:refnum<vi>)
          n68 = Unbundle By Name(w123) -> ("Target.X::4"=w120:refnum<vi>, "Target.Y::4"=w121:refnum<vi>)
          n69 = property class="DigNum (strict)"(reference=w120) -> ("Value"=w134:dbl)  [unwired: 1 in, 2 out]
          n70 = property class="DigNum (strict)"(reference=w121) -> ("Value"=w135:dbl)  [unwired: 1 in, 2 out]
          n71 = property class="DigNum (strict)"(reference=w127) -> ("Value"=w129:dbl)  [unwired: 1 in, 2 out]
          n72 = property class="DigNum (strict)"(reference=w128) -> ("Value"=w130:dbl)  [unwired: 1 in, 2 out]
          n73 = Bundle("Value"=w134, "Value"=w135) -> (w136:cluster{"Value":dbl, "Value":dbl})  [unwired: 1 in]
          n74 = Bundle("Value"=w129, "Value"=w130) -> (w137:cluster{"Value":dbl, "Value":dbl})  [unwired: 1 in]
          n75 = Bundle By Name(cluster=T14 {"Draw"=TRUE, "Target"={"x"=20.0, "y"=20.0}, "Size"={"x"=20.0, "y"=20.0}, "Angle"=1250067.0, "Color"=1250067, "Thickness"=5, "CrosshairLabel"=""} ("Crosshair"), "Draw"=TRUE, "Target"=w136, "Size"=w137, "Angle"=0.0, "Color"="Color Box") -> (w132:T14)
          n76 = call "draw crosshair imaq.vi"("Crosshair"=w132, "Bounding Rectangle"=T15 {"Left"=0, "Top"=0, "Right"=0, "Bottom"=0}, "image in"=w115) -> ("error out"=→"error out":errorcluster)  [unwired: 7 in, 1 out]
        }
      }
      frame "GetDefaultsNew" {
        n77 = call "GetDefaultXhairs.vi"("appended array 2"=w143) -> ("appended array"=→"appended array":string[], "appended array 4"=→"appended array 4":string[], "appended array 6"=→"appended array 6":string[])  [unwired: 1 out]
      }
      frame "---------- Core ----------" {
        # "Do not put any code in this frame.\n(it is a separator no-op)"
        n78 = call <vilib>:"Add State(s) to Queue__jki_lib_state_machine.vi"("State(s) in (\"\")"=w150) -> ("States Out"=w149:string)  [unwired: 14 in]
      }
      frame Default {
        w160 = 42 items=["No error", "Argument error", "Memory is full", "Out of zone", "End of file", "File already open", "Generic file I/O error", "File not found", "File permission error", "Disk is full", "Duplicate path", "Too many files open", "System feature not enabled", "Resource file not found", "Cannot add resource", "Resource not found", "Image not found", "Image memory error", "Pen does not exist", "Config type invalid", "Config token not found", "Config parse error", "Config memory error", "Bad external code format", "Bad external code offset", "External code not present", "Null window", "Destroy window error", "Null menu", "Print aborted", "Bad print record", "Print driver error", "Windows error during printing", "Memory error during printing", "Print dialog error", "Generic print error", "Invalid device refnum", "Device not found", "Device parameter error", "Device unit error", "Cannot open device", "Device call aborted", "Generic error", "Cancelled by user", "Object ID too low", "Object ID too high", "Object not in heap", "Unknown heap", "Unknown object (invalid DefProc)", "Unknown object (DefProc not in table)", "Message out of range", "Invalid (null) method", "Unknown message", "Manager call not supported", "Bad address", "Network operation in progress", "Network operation timed out", "Connection is busy", "Network attribute not supported", "Network error", "Address in use", "System out of memory", "Connection aborted", "Connection refused", "Not connected", "Already connected", "Connection closed", "Initialization error (interapplication manager)", "Bad occurrence", "Wait on unbound occurrence handler", "Occurrence queue overflow", "Datalog type conflict", "Unused", "Unrecognized type (interapplication manager)", "Memory corrupt", "Failed to make temporary DLL", "Old CIN version", "Drag socket not found", "Failed to load drop-object", "Failed to register OLE object", "Failed to release OLE object", "Format specifier type mismatch", "Unknown format specifier", "Too few format specifiers", "Too many format specifiers", "Scan failed", "Newer CIN version", "Error converting to variant", "Runtime menu error", "Password tampered", "Variant attribute not found", "Incompatible variant data type", "Event data is not available", "Event Store is not present", "Occurrence is not found", "Event Queue is not created", "Event info is not available", "Refnum passed is NULL", "Error retrieving Class GUID", "Error retrieving CoClass GUID", "Error retrieving TypeLib GUID.", "Bad built application magic bytes.", "Specific driver is different from the specific driver associated with the Logical Name.", "There is no session opened to the class driver.", "Max Error", "MAX - Error with config objects", "MAX - Error loading configuration", "MAX - Group not supported"]
        # "Current State"
        # "Do not delete, rename, or modify this frame.\n(this is used to capture unhandled states and typos)"
        # "Handle mistyped state name (developer tool)"
        n79 = call <vilib>:"Add State(s) to Queue__jki_lib_state_machine.vi"("State(s) in (\"\")"=w155) -> ("States Out"=w154:string)  [unwired: 14 in]
        n80 = Format Into String(format string="Software Exception: Unhandled State \"%s\"." ("message"), error in=w156, w151) -> (resulting string=w159:string, error out=w158:errorcluster)  [unwired: 1 in]
        n81 = call <vilib>:"Error Cluster From Error Code.vi"("show call chain? (False)"=TRUE, "error in (no error)"=w158, "error message (\"\")"=w159, "error code (0)"=w160) -> ("error out"=w157:errorcluster)  [unwired: 5 in]
      }
      frame "Initialize Core Data" {
        # "Do not delete, rename, or modify this frame.\n(this is used to determine panel behavior on exit)"
        # "originally closed?"
        # "exe?"
        # "If panel starts closed or is an EXE, then close it when we exit"
        n82 = call <vilib>:"Add State(s) to Queue__jki_lib_state_machine.vi"("State(s) in (\"\")"=w173) -> ("States Out"=w172:string)  [unwired: 14 in]
        n83 = property class="VI"() -> ("Front Panel.Open"=w169:bool)  [unwired: 2 in, 2 out]
        n84 = Not(x=w169) -> (.not. x?=w166:bool)
        n85 = property class="App"() -> ("App.Kind"=w168:T16)  [unwired: 2 in, 2 out]
        n86 = Equal?(x=w168, y=T16."Run Time System" ("Application:Kind")) -> (x = y?=w165:bool)
        n87 = control-ref of="Current VI Reference"() -> (w162:refnum<vi>)
        n88 = Or(x=w166, y=w165) -> (x .or. y?=w163:bool)
        n89 = Bundle By Name(cluster=w164, "Core.Current VI Reference"=w162, "Core.Close Panel on Exit?"=w163) -> (w171:T19)
      }
      frame "Error Handler" {
        # "Unhandled Error -- Display it"
        # "Handle any errors here.\nYou can also output any states to clean-up after errors occur"
        # "Clear error"
        n90 = call <vilib>:"General Error Handler.vi"("error in (no error)"=w175) -> ()  [unwired: 10 in, 5 out]
        n91 = call <vilib>:"Add State(s) to Queue__jki_lib_state_machine.vi"("State(s) in Front (\"\")"="/* Post Error States", "State(s) in (\"\")"=w179) -> ("States Out"=w178:string)  [unwired: 13 in]
      }
      frame "Exit" {
        # "Do not put any code in this frame.\n(No errors that occur here will be handled.)"
        n92 = call <vilib>:"Add State(s) to Queue__jki_lib_state_machine.vi"("State(s) in (\"\")"=w184) -> ("States Out"=w183:string)  [unwired: 14 in]
      }
      frame "---------- Data ----------" {
        # "Do not put any code in this frame.\n(It is a separator no-op. You can make a copy of this frame to create a new Data frame)"
        n93 = call <vilib>:"Add State(s) to Queue__jki_lib_state_machine.vi"("State(s) in (\"\")"=w188) -> ("States Out"=w187:string)  [unwired: 14 in]
      }
      frame "Data: Initialize" {
        w189 = T20 {"STOP queue"=refnum, "SuperGUI ref"=refnum}  # SuperGUI
        w190 = T21 {"Current VI Reference"=refnum, "Close Panel on Exit?"=FALSE}  # Core
        w192 = TRUE  # Your Boolean data
        # "Initialize the shift-register data, here.\n(data names are defined by what you wire into the bundle function)"
        n94 = call <vilib>:"Add State(s) to Queue__jki_lib_state_machine.vi"("State(s) in (\"\")"=w196) -> ("States Out"=w195:string)  [unwired: 14 in]
        n95 = Bundle("Core"=w190, "Your Boolean data"=w192, "active cams"="active cams", "SuperGUI"=w189) -> (w194:T19)  [unwired: 1 in]
      }
      frame "Data: Cleanup" {
        # "Cleanup any data and references, here.\n(this is called automatically, by the Macro: Exit)"
        n96 = Unbundle By Name(w197) -> ("Core.Current VI Reference"=w200:refnum<vi>)
        n97 = call <vilib>:"Add State(s) to Queue__jki_lib_state_machine.vi"("State(s) in (\"\")"=w202) -> ("States Out"=w201:string)  [unwired: 14 in]
        n98 = Close Reference(reference=w200, error in (no error)=w199) -> (error out=w198:errorcluster)
      }
      frame "---------- UI ----------" {
        # "Do not put any code in this frame.\n(It is a separator no-op. You can make a copy of this frame to create a new UI frame)"
        n99 = call <vilib>:"Add State(s) to Queue__jki_lib_state_machine.vi"("State(s) in (\"\")"=w206) -> ("States Out"=w205:string)  [unwired: 14 in]
      }
      frame "UI: Initialize" {
        # "Initialize the User Interface, here.\n(this is called automatically, by the Macro: Init)"
        n100 = call <vilib>:"Add State(s) to Queue__jki_lib_state_machine.vi"("State(s) in (\"\")"=w213) -> ("States Out"=w212:string)  [unwired: 14 in]
        n101 = call <userlib>:"Fit VI window to Largest Dec__ogtk.vi"("error in (no error)"=w210) -> ("error out"=w209:errorcluster)  [unwired: 5 in, 1 out]
        n102 = for {
          tunnel: string[] ["Point Grey Camera", "Manta Camera", "Photometrics Cam", "Basler Camera"] -> [w215] mode=indexing
          tunnel: [w214] -> w207 mode=concatenating
          n103 = call "getDevices.vi"("Device Class"=w215) -> ("All Devices"=w214:string[])
        }
        n104 = property on="Select device" class="CmbBox"("Strings[]"=w207) -> ()  [unwired: 2 in, 2 out]
      }
      frame "UI: Get Device Name" {
        # "Initialize the User Interface, here.\n(this is called automatically, by the Macro: Init)"
        n105 = call <vilib>:"Add State(s) to Queue__jki_lib_state_machine.vi"("State(s) in (\"\")"=w221) -> ("States Out"=w220:string)  [unwired: 14 in]
        n106 = First Call?() -> (First Call?: T/F=w218:bool)
        n107 = case shown="True" w218 {
          tunnel: w217 -> [w222 w224]
          tunnel: [w222 w223] -> w216
          frame False {
          }
          frame True {
            n108 = disable-structure "Get Device name from control for vi mode\nand command line arg for exe" shown="RUN_TIME_ENGINE==True" {
              disable-tunnel: w224 -> [w225 w227]
              disable-tunnel: [w225 w226] -> w223
              frame condition #0 (active) {
              }
              frame condition #1 {
                n109 = control-ref of="This Application"() -> (w235:refnum<vi>)
                n110 = property class="App"(reference=w235) -> ("App.Args"=w234:string[])  [unwired: 1 in, 2 out]
                n111 = Index Array(array=w234, index #1=1 ("index")) -> (element #1=w228:string)  [unwired: 2 in, 2 out]
                n112 = Empty String/Path?(string/path=w228) -> (empty?=w232:bool)
                n113 = Concatenate Strings(w228, "_GUI ") -> (w230:string)
                n114 = case shown="False" w232 {
                  tunnel: w228 -> [w236 _]
                  frame False {
                    n115 = local write "GUIdevice 1"(w236) -> ()
                  }
                  frame True {
                  }
                }
                n116 = control-ref of="This VI"() -> (w231:refnum<vi>)
                n117 = property class="VI"(reference=w231, error in=w227, "Front Panel.Title"=w230) -> (error out=w226:errorcluster)  [unwired: 1 out]
              }
            }
          }
        }
      }
      frame "UI: Start SuperGUI" {
        # "create stop queue for supergui and its clones"
        # "x100 abort will be dependent on caller VI\nx80 abort will be independent of caller vi, this will abort vi when labview is closed."
        # "Start SuperGUI asynchronous way"
        n118 = vi-ref "GUI_Master_subvi_reentrant_queues.vi"() -> (w239:refnum<vi>)
        n119 = property class="VI"(reference=w239) -> ("Path"=w238:path)  [unwired: 1 in, 2 out]
        n120 = control-ref of="This Application"() -> (w245:refnum<vi>)
        n121 = Open VI Reference(type specifier VI Refnum (for type only)=refnum<vi> refnum, vi path=w238, options=256) -> (vi reference=w254:refnum<vi>, error out=w253:errorcluster)  [unwired: 3 in]
        n122 = Create User Event(user event datatype=T17 {"EventEnum"=enum."new data", "Device name"="Device name"} ("New Event"), error in=w241) -> (user event=w242:refnum<user-event>, error out=w248:errorcluster)
        "tcp data event" <- w242
        n123 = control-ref of="This VI"() -> (w244:refnum<vi>)
        n124 = register-events(w242) -> ()  [unwired: 2 in, 2 out]
        n125 = call "supergui create stop queue.vi"() -> ("STOP Queue out"=w250:refnum<queue>)  [unwired: 11 in]
        n126 = Current VI's Menubar() -> (w243:refnum<k9>)
        n127 = call-by-ref "Start Asynchronous Call"(reference=w254, error in=w253, "STOP Queue in"=w250, "This Application"=w245, 8:"error in (no error)"=w248, "tcp data event"=w242, "Caller menu reference"=w243, "Caller VI ref"=w244) -> (reference out=w237:refnum<vi>, error out=w240:errorcluster)  [unwired: 5 in, 1 out]
        n128 = Bundle By Name(cluster=w247, "SuperGUI.SuperGUI ref"=w237, "SuperGUI.STOP queue"=w250) -> (w246:T19)
        n129 = call <vilib>:"Add State(s) to Queue__jki_lib_state_machine.vi"("State(s) in (\"\")"=w256) -> ("States Out"=w255:string)  [unwired: 14 in]
      }
      frame "UI: Stop SuperGUI" {
        # "Stop Supergui Clone and wait until it exit properly"
        n130 = call <vilib>:"Add State(s) to Queue__jki_lib_state_machine.vi"("State(s) in (\"\")"=w264) -> ("States Out"=w263:string)  [unwired: 14 in]
        n131 = Unbundle By Name(w259) -> ("SuperGUI.SuperGUI ref"=w261:refnum<vi>, "SuperGUI.STOP queue"=w260:refnum<queue>)
        n132 = Release Queue(queue=w260, error in (no error)=w258) -> (error out=w262:errorcluster)  [unwired: 1 in, 2 out]
        n133 = call-by-ref "Wait On Asynchronous Call"(reference=w261, error in=w262) -> ("error out"=w257:errorcluster)  [unwired: 11 in, 2 out]
      }
      frame "UI: Cursor Set" {
        # "Argument"
        # "Set and Unset Cursor Busy.\n(Usage: \"UI: Cursor Set >> Busy|Idle\")"
        n134 = call <vilib>:"Add State(s) to Queue__jki_lib_state_machine.vi"("State(s) in (\"\")"=w270) -> ("States Out"=w269:string)  [unwired: 14 in]
        n135 = case shown="\"Idle\", Default" w265 {
          tunnel: w267 -> [w272 w274]
          tunnel: [w271 w273] -> w266
          frame "Idle", Default {
            n136 = call <vilib>:"Unset Busy.vi"("error in (no error)"=w272) -> ("error out"=w271:errorcluster)  [unwired: 10 in]
          }
          frame "Busy" {
            n137 = call <vilib>:"Set Busy.vi"("error in (no error)"=w274) -> ("error out"=w273:errorcluster)  [unwired: 9 in, 1 out]
          }
        }
      }
      frame "UI: Front Panel State" {
        # "Argument"
        # "Set Front Panel Open or Closed\n(Usage: \"UI: Front Panel State >> Open|Close\")"
        n138 = call <vilib>:"Add State(s) to Queue__jki_lib_state_machine.vi"("State(s) in (\"\")"=w281) -> ("States Out"=w280:string)  [unwired: 14 in]
        n139 = Unbundle By Name(w277) -> ("Core.Current VI Reference"=w276:refnum<vi>)
        n140 = case shown="\"Open\", Default" w275 {
          tunnel: w279 -> [w285 w298]
          tunnel: [w287 w299] -> w278
          tunnel: w276 -> [w286 w296]
          frame "Open", Default {
            n141 = property class="VI"(reference=w286, error in=w285) -> (reference out=w283:refnum<vi>, error out=w284:errorcluster, "Front Panel.Open"=w282:bool)
            n142 = case shown="False" w282 {
              tunnel: [w290 w293] -> w287
              tunnel: w284 -> [w289 w293]
              tunnel: w283 -> [w288 _]
              frame False {
                n143 = invoke class="VI" method="FP.Open"(reference=w288, error in=w289, "Activate"=TRUE, "State"=T18."Standard") -> (error out=w290:errorcluster)  [unwired: 1 in, 4 out]
              }
              frame True {
              }
            }
          }
          frame "Close" {
            n144 = property class="VI"(reference=w296, error in=w298) -> (reference out=w295:refnum<vi>, error out=w297:errorcluster, "Front Panel.Open"=w294:bool)
            n145 = case shown="True" w294 {
              tunnel: [w300 w303] -> w299
              tunnel: w297 -> [w300 w302]
              tunnel: w295 -> [_ w301]
              frame False {
              }
              frame True {
                n146 = invoke class="VI" method="FP.Close"(reference=w301, error in=w302) -> (error out=w303:errorcluster)  [unwired: 1 in, 2 out]
              }
            }
          }
        }
      }
      frame "---------- Macro ----------" {
        # "Do not put any code in this frame.\n(It is a separator no-op. You can make a copy of this frame to create a new Macro frame)"
        n147 = call <vilib>:"Add State(s) to Queue__jki_lib_state_machine.vi"("State(s) in (\"\")"=w307) -> ("States Out"=w306:string)  [unwired: 14 in]
      }
      frame "Macro: Initialize" {
        # "Initialization Macro\n(This is called once, when the VI starts)"
        n148 = call <vilib>:"Add State(s) to Queue__jki_lib_state_machine.vi"("State(s) in Front (\"\")"="Data: Initialize\nInitialize Core Data\nUI: Initialize\nUI: Get Device Name\nUI: Start SuperGUI\nUI: Front Panel State >> Open", "State(s) in (\"\")"=w312) -> ("States Out"=w311:string)  [unwired: 13 in]
      }
      frame "Macro: Exit" {
        # "Exit Macro\n(This is called once, when the VI exits)"
        n149 = Unbundle By Name(w320) -> ("Core.Close Panel on Exit?"=w319:bool)
        n150 = Select(t="UI: Front Panel State >> Close", s=w319, f="") -> (s? t:f=w316:string)
        n151 = call <vilib>:"Add State(s) to Queue__jki_lib_state_machine.vi"("State(s) in Front (\"\")"="UI: Stop SuperGUI" ("State(s) in Front (\"\")"), "State(s) in (\"\")"=w316, "State(s) at Back (\"\")"="Data: Cleanup\nExit") -> ("States Out"=w314:string)  [unwired: 12 in]
        n152 = call <vilib>:"Add State(s) to Queue__jki_lib_state_machine.vi"("State(s) in Front (\"\")"=w314, "State(s) in (\"\")"=w323) -> ("States Out"=w322:string)  [unwired: 13 in]
      }
      frame "---------- New Category ----------" {
        # "Template Separator\n(You can make a copy of, or modify, this frame)"
        n153 = call <vilib>:"Add State(s) to Queue__jki_lib_state_machine.vi"("State(s) in (\"\")"=w327) -> ("States Out"=w326:string)  [unwired: 14 in]
      }
      frame "New Category: 1" {
        # "Your code here.\n(You can make a copy of, or modify, this frame)"
        n154 = call <vilib>:"Add State(s) to Queue__jki_lib_state_machine.vi"("State(s) in (\"\")"=w331) -> ("States Out"=w330:string)  [unwired: 14 in]
      }
      frame "New Category: 2" {
        # "Your code here.\n(You can make a copy of, or modify, this frame)"
        n155 = call <vilib>:"Add State(s) to Queue__jki_lib_state_machine.vi"("State(s) in (\"\")"=w335) -> ("States Out"=w334:string)  [unwired: 14 in]
      }
    }
  }
